vi "UseCaseDiagramGraph_SetModifiedAttributes.vi"(0 "reference in":refnum<class "UseCaseDiagramGraph.lvclass">, 2 "Attributes":T1, 3 "Only unlock data? (F)":bool, 4 "Unlock data if error? (T)":bool=TRUE, 5 "error in (no error)":errorcluster, 7 "Update data even if error? (F)":bool) -> (14 "reference out":refnum<class "UseCaseDiagramGraph.lvclass">, 19 "error out":errorcluster)   [LabVIEW 2020, in "UseCaseDiagramGraph.lvclass"]
doc: "This VI overwrites the attributes associated with the UseCaseDiagramGraph object reference and unlocks it for write access. If error in is set, the object is unlocked but its data will not be modified.\n\nIn order to use this VI, you must first successfully lock the object's data using the UseCaseDiagramGraph GetAttributesToModify VI.\n\n[GOOP 2.0.15]"
uses:
  <resource>/Framework/Providers/Open_GDS/UML/UseCaseDiagramGraph_class/UseCaseDiagramGraph.lvclass
  <vilib>/addons/_goop3.llb/3GOOPStates.ctl
  <resource>/Framework/Providers/Open_GDS/UML/UseCaseDiagramGraph_class/protected/ObjectAttributes.ctl
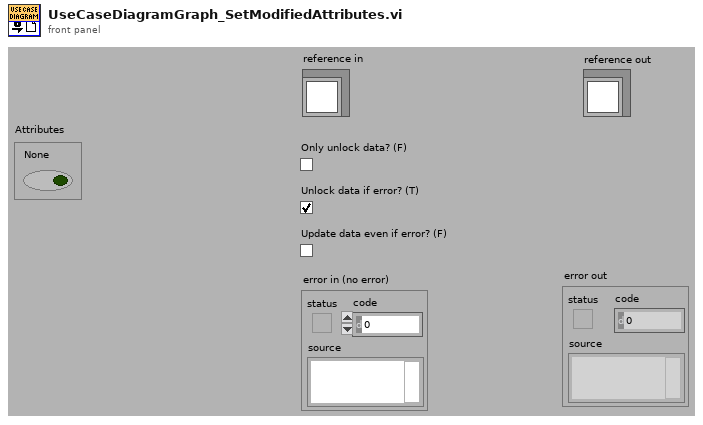
[diagram p1: front panel]
types:
  T1 = typedef "UseCaseDiagramGraph.lvclass/ObjectAttributes.ctl" = cluster{"None":bool}
  T2 = typedef "Graph.lvclass/ObjectReference.ctl" = refnum<k1>
  T3 = typedef "3GOOPStates.ctl" = enum16{"Set", "Get", "New", "Delete", "Clear", "Test and get", "Unlock data", "Information", "Look up existing", "New or look up existing", "Test and get shared", "Get shared", "Set shared", "Unlock shared", "Find dynamic method", "Register dynamic method", "Preload dynamic method", "Probe", "Cast to more generic", "Cast to more specific"}
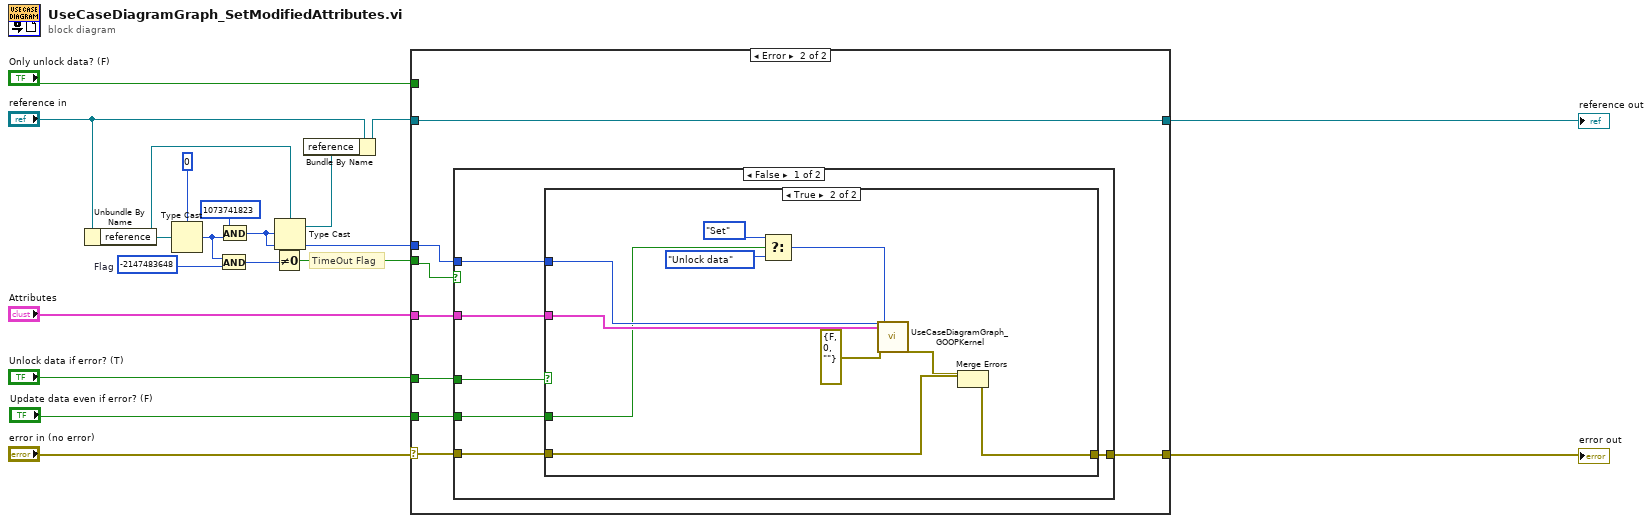
[diagram p0: block diagram]
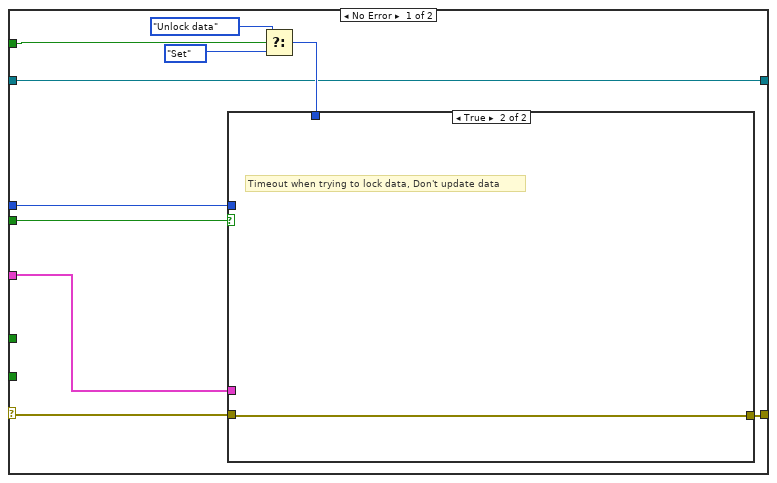
[diagram p2: hidden frame]
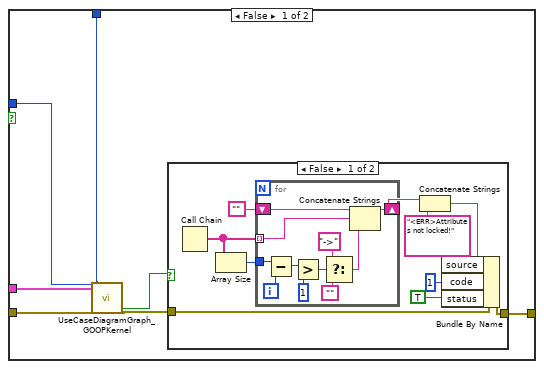
[diagram p3: hidden frame]
diagram:
  w8 = -2147483648  # Flag
  # "TimeOut Flag"
  n1 = Unbundle By Name("reference in") -> ("reference"=w10:T2)
  n2 = Type Cast(type=0, x=w10) -> (*(type *) &x=w9:i32)
  n3 = And(x=w9, y=w8) -> (x .and. y?=w7:i32)
  n4 = And(x=1073741823 ("x .and. y?"), y=w9) -> (x .and. y?=w5:i32)
  n5 = Not Equal To 0?(x=w7) -> (x != 0?=w4:bool)
  n6 = Type Cast(type=w10, x=w5) -> (*(type *) &x=w6:T2)
  n7 = Bundle By Name(cluster="reference in", "reference"=w6) -> (w3:refnum<class "UseCaseDiagramGraph.lvclass">)
  n8 = case shown="Error" "error in (no error)" {
    selector: "error in (no error)" -> [w27 w63]
    tunnel: [w19 w66] -> w14
    tunnel: "Attributes" -> [w23 w65]
    tunnel: [w22 w59] -> w13
    tunnel: w3 -> [w19 w66]
    tunnel: "Only unlock data? (F)" -> [w28 _]
    tunnel: "Unlock data if error? (T)" -> [_ w64]
    tunnel: w5 -> [w21 w61]
    tunnel: w4 -> [w20 w60]
    tunnel: "Update data even if error? (F)" -> [_ w62]
    frame No Error {
      n9 = Select(t=3GOOPStates."Unlock data" ("Action"), s=w28, f=3GOOPStates."Set" ("Action")) -> (s? t:f=w24:T3)
      n10 = case shown="True" w20 {
        tunnel: w27 -> [w35 w58]
        tunnel: w24 -> [w34 _]
        tunnel: w23 -> [w33 _]
        tunnel: [w31 w58] -> w22
        tunnel: w21 -> [w29 _]
        frame False {
          n11 = call <resource>:"UseCaseDiagramGraph_GOOPKernel.vi"("Ref in"=w29, "Data in"=w33, "error in (no error)"=w35, "Action"=w34) -> ("Data locked?"=w30:bool, "error out"=w32:errorcluster)  [unwired: 11 in, 11 out]
          n12 = case shown="False" w30 {
            tunnel: w32 -> [w40 w57]
            tunnel: [w41 w57] -> w31
            frame False {
              n13 = Call Chain() -> (call chain=w36:string[])
              n14 = Array Size(array=w36) -> (size(s)=w44:i32)
              n15 = for {
                shift-right: [w50] -> w43
                shift-left: "" -> [w52]
                tunnel: w36 -> [w51] mode=indexing
                tunnel: w44 -> [w56]
                i -> [w55]
                n16 = Subtract(x=w56, y=w55) -> (x-y=w54:i32)
                n17 = Greater?(x=w54, y=1) -> (0:w47:bool)
                n18 = Select(t="->", s=w47, f="") -> (s? t:f=w46:string)
                n19 = Concatenate Strings(w52, w51, w46) -> (w50:string)
              }
              n20 = Concatenate Strings(w43, "<ERR>Attributes not locked!" ("Bundle Element")) -> (w39:string)
              n21 = Bundle By Name(cluster=w40, "source"=w39, "code"=1, "status"=TRUE) -> (w41:errorcluster)
            }
            frame True {
            }
          }
        }
        frame True {
          # "Timeout when trying to lock data, Don't update data"
        }
      }
    }
    frame Error {
      n22 = case shown="False" w60 {
        tunnel: w64 -> [w72 _]
        tunnel: w63 -> [w71 w84]
        tunnel: [w70 w84] -> w59
        tunnel: w61 -> [w69 _]
        tunnel: w65 -> [w68 _]
        tunnel: w62 -> [w67 _]
        frame False {
          n23 = case shown="True" w72 {
            tunnel: w71 -> [w73 w82]
            tunnel: [w73 w83] -> w70
            tunnel: w69 -> [_ w78]
            tunnel: w68 -> [_ w77]
            tunnel: w67 -> [_ w74]
            frame False {
            }
            frame True {
              n24 = Select(t=3GOOPStates."Set" ("Action"), s=w74, f=3GOOPStates."Unlock data" ("Action")) -> (s? t:f=w79:T3)
              n25 = call <resource>:"UseCaseDiagramGraph_GOOPKernel.vi"("Ref in"=w78, "Data in"=w77, "error in (no error)"=errorcluster {"status"=FALSE, "code"=0, "source"=""}, "Action"=w79) -> ("error out"=w75:errorcluster)  [unwired: 11 in, 12 out]
              n26 = Merge Errors(w82, w75) -> (w83:errorcluster)
            }
          }
        }
        frame True {
          # "Timeout when trying to lock data, Don't update data"
        }
      }
    }
  }
  "error out" <- w13
  "reference out" <- w14
